vi "FGV_SQL_TEXT_records_display.vi"(4 "front_panel_reference":refnum<vi>, 6 "SQL_listbox_reference":refnum<vi>, 7 "options":T1, 8 "error_in":errorcluster, 11 "input":variant) -> (0 "error_out":errorcluster)   [LabVIEW 2019]
uses:
  FGV_SQL_TEXT_records_display.ctl
  SQL_TEXT_all_info.ctl
  <vilib>/addons/database/_DB Variant To Data/Database Variant To Data.xnode
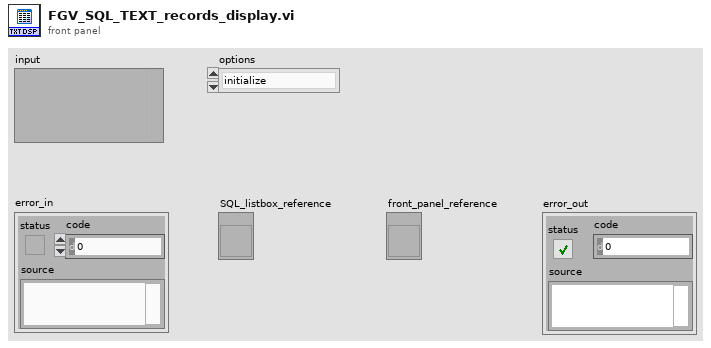
[diagram p1: front panel]
types:
  T1 = typedef "FGV_SQL_TEXT_records_display.ctl" = enum16{"initialize", "set", "clear"}
  T2 = typedef "SQL_TEXT_all_info.ctl" = cluster{"headers":string[], "values":string[][]}
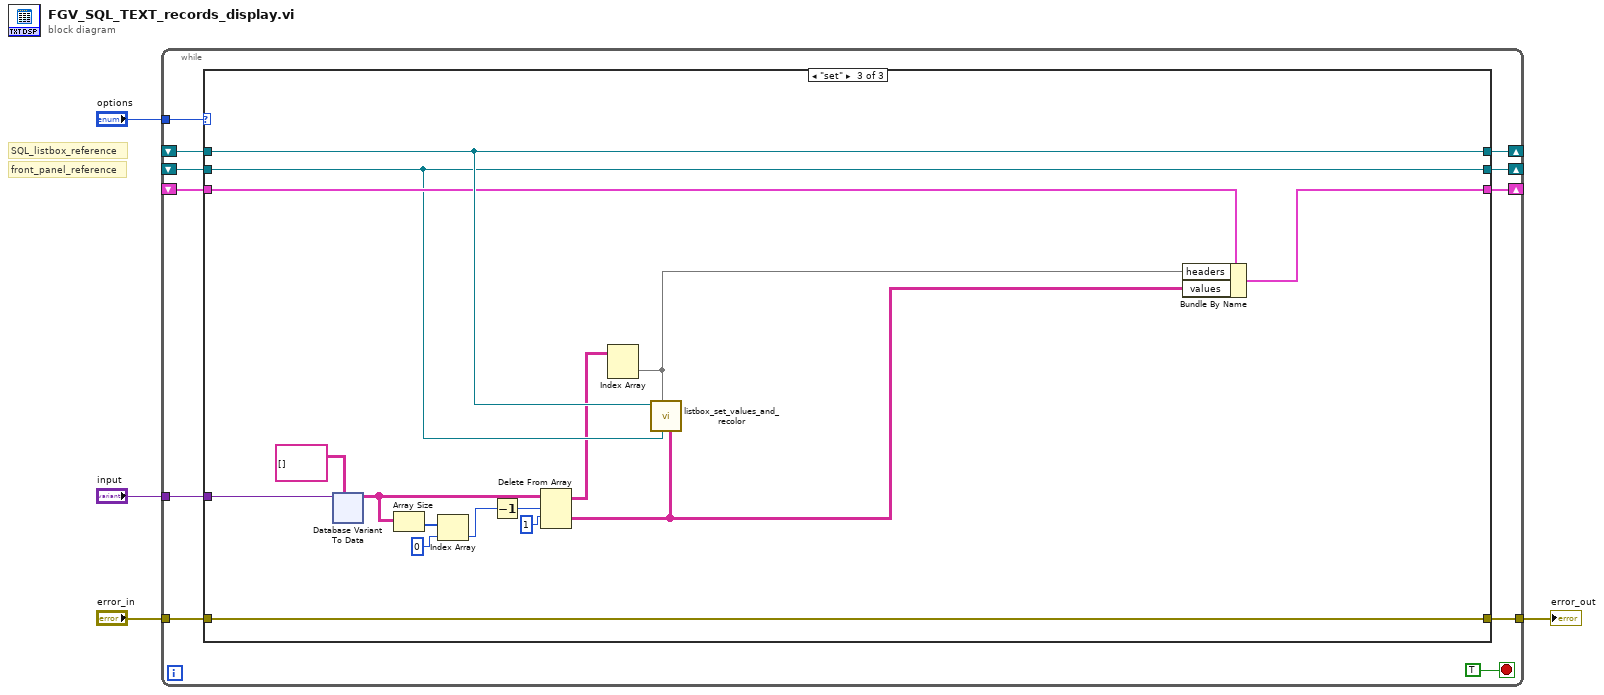
[diagram p0: block diagram]
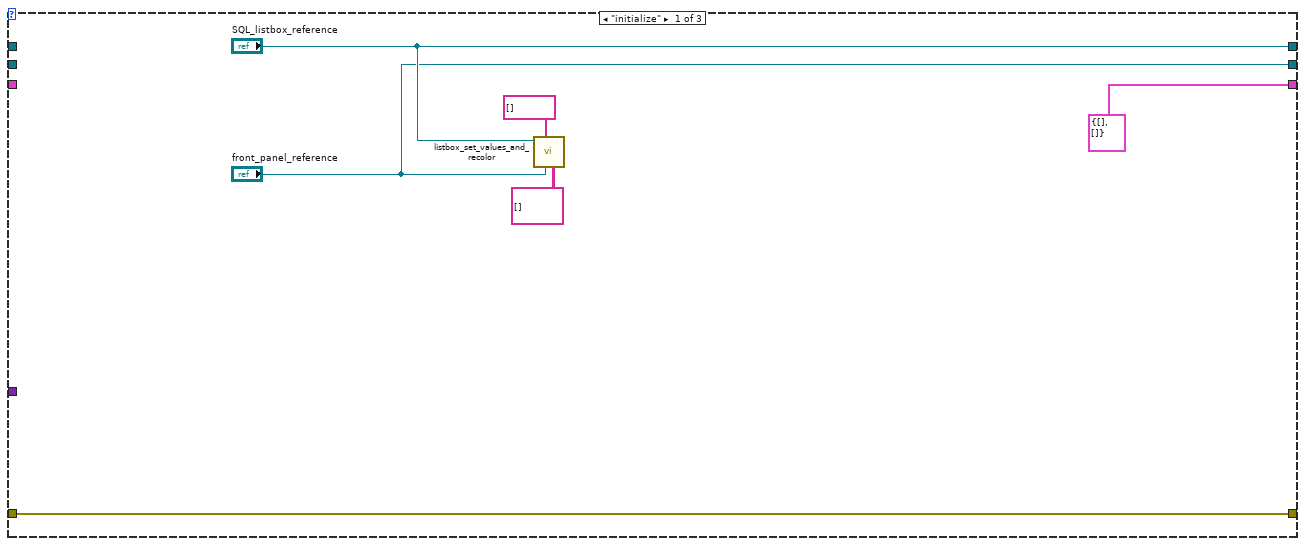
[diagram p2: hidden frame]
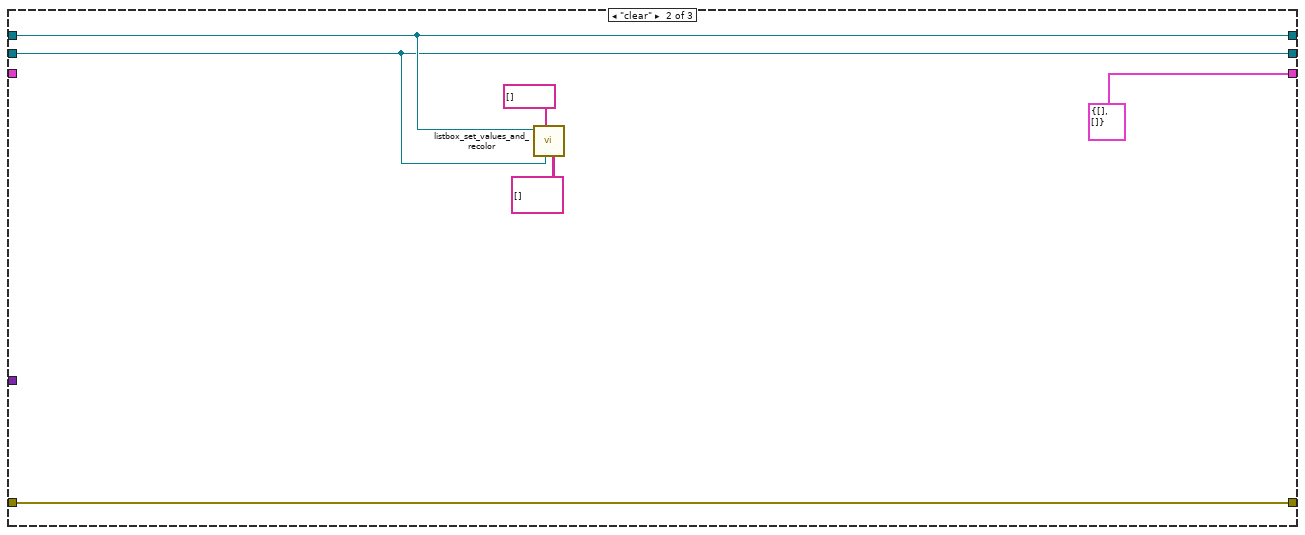
[diagram p3: hidden frame]
diagram:
  # "front_panel_reference"
  # "SQL_listbox_reference"
  n1 = while {
    tunnel: "options" -> [w14]
    tunnel: [w13] -> w4
    tunnel: "error_in" -> [w12]
    shift-right: [w11] -> _
    shift-left: _ -> [w10]
    shift-right: [w9] -> _
    shift-left: _ -> [w8]
    tunnel: "input" -> [w7]
    shift-right: [w6] -> _
    shift-left: _ -> [w5]
    stop <- TRUE stop-if-true
    n2 = case shown="\"set\"" w14 {
      tunnel: [w21 w27 w41] -> w13
      tunnel: w12 -> [w21 w27 w41]
      tunnel: [T2 {"headers"=[], "values"=[]} ("SQL_selection") T2 {"headers"=[], "values"=[]} ("SQL_selection") w38] -> w11
      tunnel: w10 -> [_ _ w39]
      tunnel: ["SQL_listbox_reference" w23 w40] -> w9
      tunnel: w8 -> [_ w23 w40]
      tunnel: w7 -> [_ _ w42]
      tunnel: ["front_panel_reference" w22 w37] -> w6
      tunnel: w5 -> [_ w22 w37]
      frame "initialize" {
        n3 = call "listbox_set_values_and_recolor.vi"("item_names"=string[][] [], "front_panel_reference"="front_panel_reference", "column_names"=string[] [], "multicolumn_listbox_reference_in"="SQL_listbox_reference") -> ()  [unwired: 6 in, 2 out]
      }
      frame "clear" {
        n4 = call "listbox_set_values_and_recolor.vi"("item_names"=string[][] [], "front_panel_reference"=w22, "column_names"=string[] [], "multicolumn_listbox_reference_in"=w23) -> ()  [unwired: 6 in, 2 out]
      }
      frame "set" {
        n5 = xnode "Database Variant To Data"("database variant"=w42, "type"=string[][] []) -> ("data"=w35:string[][])  [unwired: 1 in, 1 out]
        n6 = Array Size(array=w35) -> (size(s)=w34:i32[])
        n7 = Index Array(array=w34, index=0) -> (element=w32:i32)
        n8 = Decrement(x=w32) -> (x-1=w31:i32)
        n9 = Delete From Array(array=w35, length=w31, index (row)=1) -> (deleted portion=w30:string[][], array with subset deleted=w29:string[][])  [unwired: 1 in]
        n10 = Index Array(array=w29) -> (element=w28:string[])  [unwired: 2 in]
        n11 = call "listbox_set_values_and_recolor.vi"("item_names"=w30, "front_panel_reference"=w37, "column_names"=w28, "multicolumn_listbox_reference_in"=w40) -> ()  [unwired: 6 in, 2 out]
        n12 = Bundle By Name(cluster=w39, "headers"=w28, "values"=w30) -> (w38:T2)
      }
    }
  }
  "error_out" <- w4
